vi "Read.vi"(8 "error in (no error)":errorcluster, 11 "object in":refnum<class "Modbus-Instr.lvclass">) -> (0 "error out":errorcluster, 2 "Data":dbl[](array[numeric]), 3 "object out":refnum<class "Modbus-Instr.lvclass">)   [LabVIEW 2021, in "Modbus-Instr.lvclass"]
doc: "Read converted data from modbus Reg"
uses:
  Modbus-Instr.lvclass
  Modbus-Instr.lvclass/Modbus-Instr.ctl
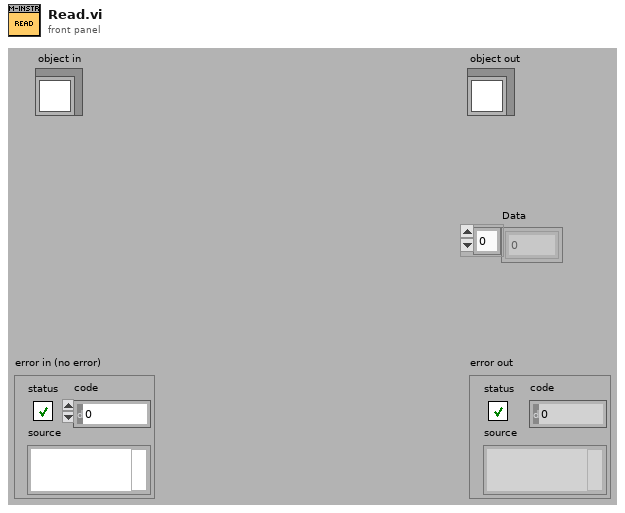
[diagram p1: front panel]
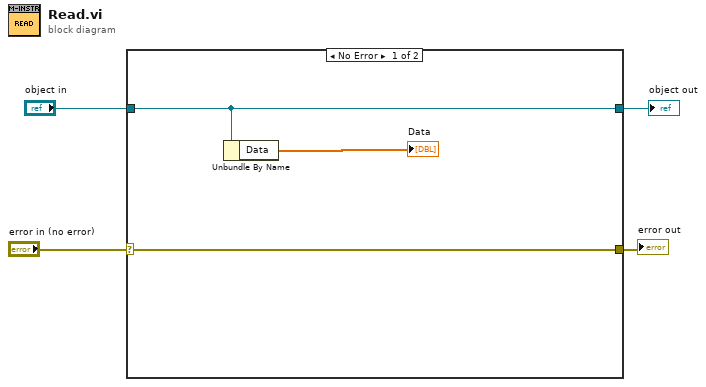
[diagram p0: block diagram]
diagram:
  n1 = case shown="No Error" "error in (no error)" {
    selector: "error in (no error)" -> [w7 w9]
    tunnel: [w7 w9] -> w3
    tunnel: [w6 w8] -> w1
    tunnel: "object in" -> [w6 w8]
    frame No Error {
      n2 = Unbundle By Name(w6) -> ("Data"=→"Data":dbl[])
    }
    frame Error {
    }
  }
  "error out" <- w3
  "object out" <- w1
